vi "acquisitionTEST.vi"   [LabVIEW 2015]
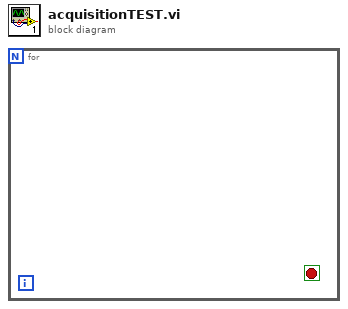
[diagram p0: block diagram]
diagram:
  n1 = for {
    stop <- _ stop-if-true
  }
